vi "Measurement Logic.vi"() -> ()   [LabVIEW 2023, in "NIDCPowerSourceDCVoltage.lvlib"]
uses:
  NIDCPowerSourceDCVoltage.lvlib
  <vilib>/Plug-In SDKs/Clients/Session Management V1/Session Reservation/Session Reservation.lvclass
  <vilib>/Plug-In SDKs/Measurements/Measure Call Context/Measure Call Context.lvclass
  <vilib>/Plug-In SDKs/Sessions/niDCPower/NI Session Management niDCPower.lvlib
  <vilib>/Plug-In SDKs/Clients/Discovery V1/NI Discovery V1 Client.lvlib
  logmeasurement_client/logmeasurement_client.lvlib
  Measurement Configuration.ctl
  Measurement Results.ctl
  <vilib>/gRPC/Generated APIs/ni/measurementlink/discovery/v1/RPC Messages/ni_measurementlink_discovery_v1_ResolveServiceRequest.ctl
  <vilib>/gRPC/Generated APIs/ni/measurementlink/discovery/v1/ni.measurementlink.discovery.v1.api.lvlib
panel:
  in  "error in":errorcluster
  in  "request data":T1
  out "error out":errorcluster
  out "measure call context out":refnum<class "Measure Call Context.lvclass">
  in  "measure call context in":refnum<class "Measure Call Context.lvclass">
  out "measurement results":T2
  in  "measurement configuration":T3={"pin_names"=[], "voltage_level"=6.0, "voltage_level_range"=6.0, "current_limit"=0.01, "current_limit_range"=0.01, "source_delay"=0.0}
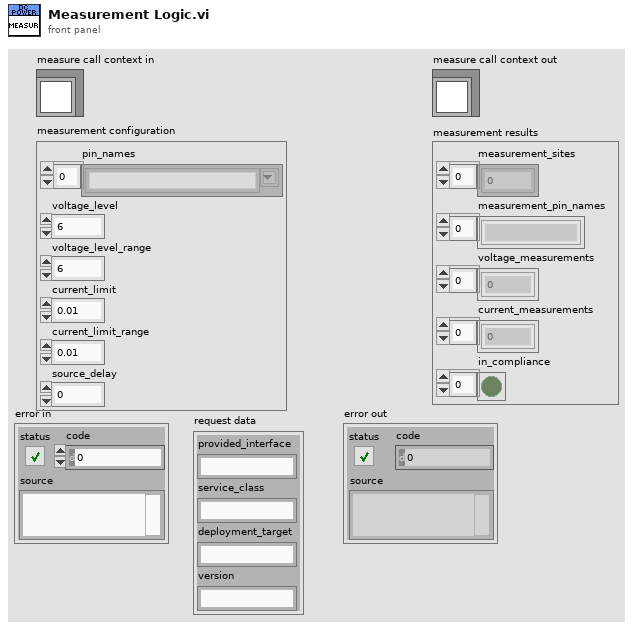
[diagram p1: front panel]
types:
  T1 = typedef "ni.measurementlink.discovery.v1.api.lvlib/ni_measurementlink_discovery_v1_ResolveServiceRequest.ctl" = cluster{"provided_interface":string, "service_class":string, "deployment_target":string, "version":string}
  T2 = typedef "NIDCPowerSourceDCVoltage.lvlib/Measurement Results.ctl" = cluster{"measurement_sites":i32[], "measurement_pin_names":string[], "voltage_measurements":dbl[], "current_measurements":dbl[], "in_compliance":bool[]}
  T3 = typedef "NIDCPowerSourceDCVoltage.lvlib/Measurement Configuration.ctl" = cluster{"pin_names":string[], "voltage_level":dbl, "voltage_level_range":dbl, "current_limit":dbl, "current_limit_range":dbl, "source_delay":dbl}
  T4 = typedef "ni.measurementlink.discovery.v1.api.lvlib/ni_measurementlink_discovery_v1_ServiceLocation.ctl" = cluster{"location":string, "insecure_port":string, "ssl_authenticated_port":string}
  T5 = typedef "NI Session Management niDCPower.lvlib/Connection with Session.ctl" = cluster{"connection":T6, "session":refnum<k15>}
  T6 = typedef "NI Session Management V1 Client.lvlib/Session Reservation.lvclass/Connection.ctl" = cluster{"pin or relay name":string, "site":i32, "instrument type id":string, "channel":string}
  T7 = typedef "grpc-lvsupport-release.lvlib/grpcId.ctl" = u64
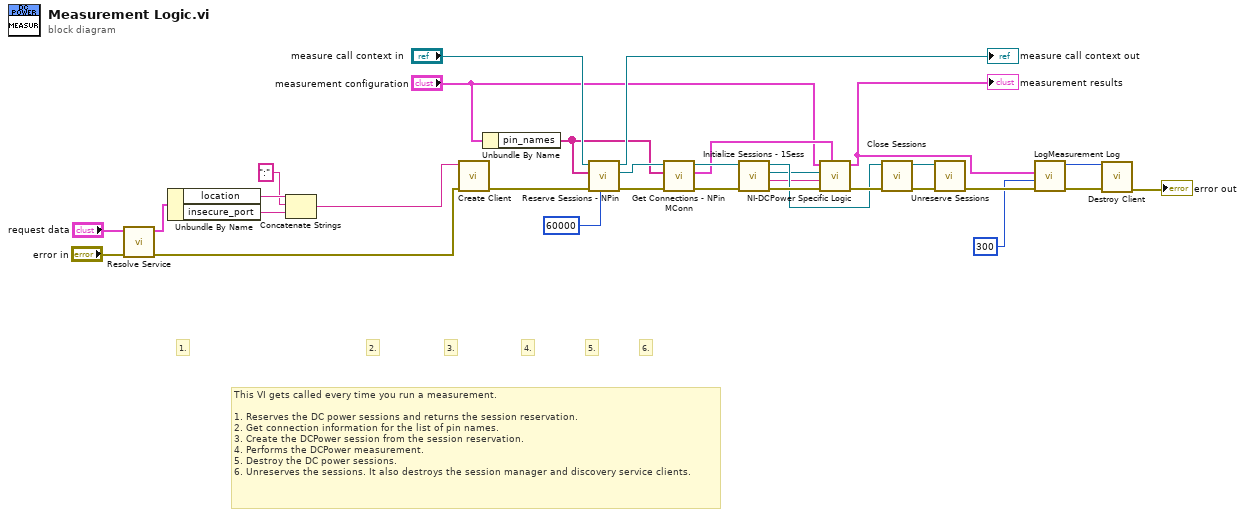
[diagram p0: block diagram]
diagram:
  # "6."
  # "This VI gets called every time you run a measurement.\n\n1. Reserves the DC power sessions and returns the session reservation.\n2. Get connection information for the list of pin names.\n3. Create the DCPower session from the session reservation.\n4. Performs the DCPower measurement.\n5. Destroy the DC power sessions.\n6. Unreserves the sessions. It also destroys the session manager and discovery service clients."
  # "5."
  # "4."
  # "3."
  # "2."
  # "1."
  n1 = call <vilib>:"Resolve Service.vi"("error in"="error in", "request data"="request data") -> ("error out"=w5:errorcluster, "response data"=w13:T4)  [unwired: 8 in]
  n2 = Unbundle By Name(w13) -> ("location"=w12:string, "insecure_port"=w10:string)
  n3 = Concatenate Strings(w12, ":" ("string"), w10) -> (w6:string)
  n4 = call "Create Client.vi"("error in"=w5, "address"=w6) -> ("error out"=w4:errorcluster)  [unwired: 8 in, 1 out]
  n5 = Unbundle By Name("measurement configuration") -> ("pin_names"=w21:string[])
  n6 = call <vilib>:"Reserve Sessions - NPin.vi"("timeout (ms)"=60000, "error in"=w4, "pin or relay names"=w21, "measurement context in"="measure call context in") -> ("error out"=w24:errorcluster, "session reservation out"=w22:refnum<class "Session Reservation.lvclass">, "measurement context out"=→"measure call context out":refnum<class "Measure Call Context.lvclass">)  [unwired: 5 in]
  n7 = call <vilib>:"Get Connections - NPin MConn.vi"("error in"=w24, "pin or relay names"=w21, "session reservation in"=w22) -> ("error out"=w23:errorcluster, "connections"=w19:T5[], "session reservation out"=w20:refnum<class "Session Reservation.lvclass">)  [unwired: 6 in]
  n8 = call <vilib>:"Initialize Sessions - 1Sess.vi"("error in"=w23, "session reservation in"=w20) -> ("error out"=w32:errorcluster, "channel list"=w17:string, "session"=w18:refnum<k15>, "session reservation out"=w28:refnum<class "Session Reservation.lvclass">)  [unwired: 6 in]
  n9 = call "NI-DCPower Specific Logic.vi"("connections"=w19, "error in"=w32, "channel list"=w17, "instrument handle"=w18, "Measurement Configuration"="measurement configuration") -> ("error out"=w31:errorcluster, "Measurement Results"=w7:T2)  [unwired: 4 in, 1 out]
  "measurement results" <- w7
  n10 = call <vilib>:"Close Sessions.vi"("error in"=w31, "session reservation in"=w28) -> ("error out"=w30:errorcluster, "session reservation out"=w29:refnum<class "Session Reservation.lvclass">)  [unwired: 8 in]
  n11 = call <vilib>:"Unreserve Sessions.vi"("error in"=w30, "session reservation in"=w29) -> ("error out"=w9:errorcluster)  [unwired: 9 in]
  n12 = call "LogMeasurement Log.vi"("error in"=w9, "timeout (ms)"=300, "Request Data"=w7) -> ("error out"=w1:errorcluster, "gRPC ID out"=w3:T7)  [unwired: 6 in, 1 out]
  n13 = call "Destroy Client.vi"("error in"=w1, "gRPC ID"=w3) -> ("error out"=→"error out":errorcluster)  [unwired: 9 in]
